vi "Find Hail Intersection (XY).vi"(9 "test area":cluster{"min":u64, "max":u64, "z":u64}, 10 "h2":T1, 11 "h1":T1) -> (3 "collide in test area in future":bool)   [LabVIEW 2022 SP3]
panel:
  out "y":dbl
  out "x":dbl
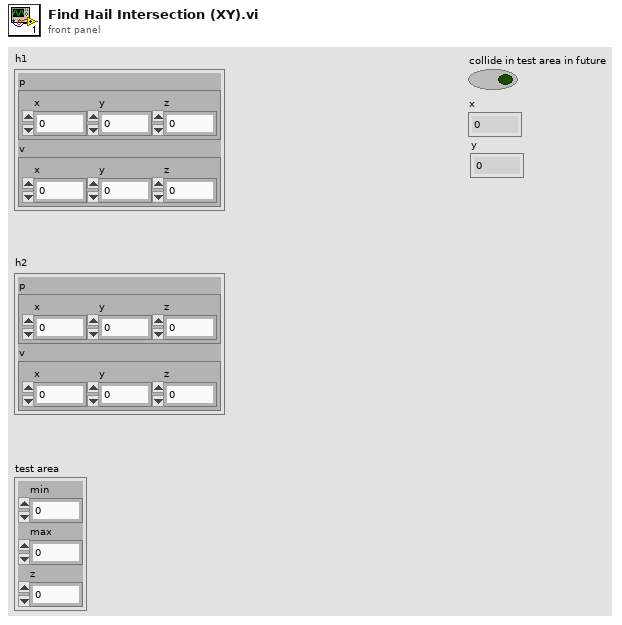
[diagram p1: front panel]
types:
  T1 = cluster{"p":cluster{"x":u64, "y":u64, "z":u64}, "v":cluster{"x":i64, "y":i64, "z":i64}}
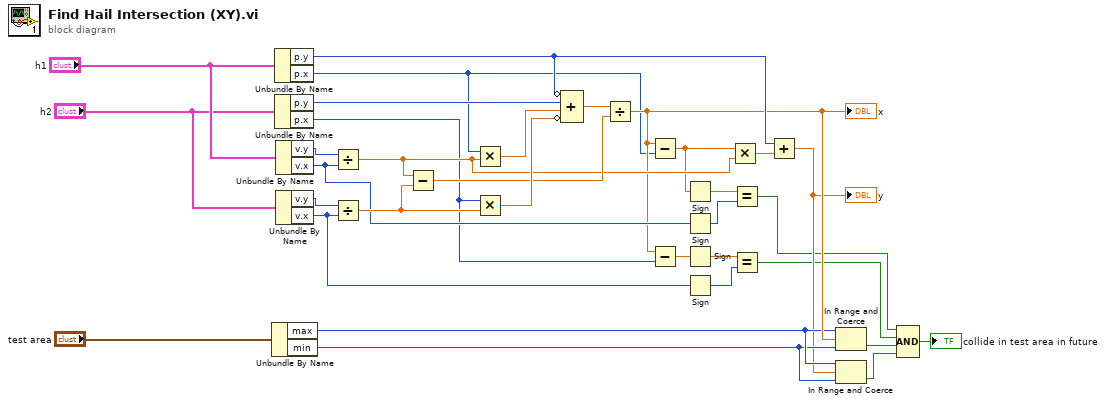
[diagram p0: block diagram]
diagram:
  n1 = Unbundle By Name("test area") -> ("max"=w12:u64, "min"=w11:u64)
  n2 = Unbundle By Name("h1") -> ("p.y"=w31:u64, "p.x"=w2:u64)
  n3 = Unbundle By Name("h2") -> ("p.y"=w32:u64, "p.x"=w1:u64)
  n4 = Unbundle By Name("h1") -> ("v.y"=w30:i64, "v.x"=w16:i64)
  n5 = Unbundle By Name("h2") -> ("v.y"=w29:i64, "v.x"=w18:i64)
  n6 = Divide(x=w30, y=w16) -> (x/y=w23:dbl)
  n7 = Divide(x=w29, y=w18) -> (x/y=w28:dbl)
  n8 = Subtract(x=w23, y=w28) -> (x-y=w24:dbl)
  n9 = Multiply(x=w2, y=w23) -> (x*y=w27:dbl)
  n10 = Multiply(x=w1, y=w28) -> (x*y=w26:dbl)
  n11 = Compound Arithmetic op=ADD(invert w31, w32, w27, invert w26) -> (w25:dbl)
  n12 = Divide(x=w25, y=w24) -> (x/y=w13:dbl)
  "x" <- w13
  n13 = Subtract(x=w13, y=w2) -> (x-y=w21:dbl)
  n14 = Subtract(x=w13, y=w1) -> (x-y=w19:dbl)
  n15 = Sign(1:w21) -> (0:w20:dbl)
  n16 = Sign(1:w16) -> (0:w15:i64)
  n17 = Sign(1:w19) -> (0:w17:dbl)
  n18 = Sign(1:w18) -> (0:w14:i64)
  n19 = Multiply(x=w21, y=w23) -> (x*y=w22:dbl)
  n20 = Equal?(x=w20, y=w15) -> (x = y?=w6:bool)
  n21 = Equal?(x=w17, y=w14) -> (x = y?=w7:bool)
  n22 = Add(x=w31, y=w22) -> (x+y=w10:dbl)
  "y" <- w10
  n23 = In Range and Coerce(upper limit=w12, x=w13, lower limit=w11) -> (In Range?=w8:bool)  [unwired: 1 out]
  n24 = In Range and Coerce(upper limit=w12, x=w10, lower limit=w11) -> (In Range?=w9:bool)  [unwired: 1 out]
  n25 = Compound Arithmetic op=AND(w6, w7, w8, w9) -> (→"collide in test area in future":bool)
